vi "FPGA_DIOWriteOutputEnable.vi"(8 "error in (no error)":errorcluster, 10 "OutputEnable":u32, 11 "DIODeviceRef In":T1) -> (0 "error out":errorcluster, 3 "DIODeviceRef Out":T1)   [LabVIEW 2017]
uses:
  <vilib>/Rock Robotics/SystemInterfaces/DIO/FPGA_DIODevRef.ctl
  <vilib>/Rock Robotics/SystemInterfaces/System/FPGA_SystemFPGA Ref Global.vi
  <vilib>/Utility/error.llb/Error Cluster From Error Code.vi
  <vilib>/rvi/errors/niLvFpgaAdjustHostInterfaceError.vi
  <vilib>/rvi/interface/nirviReadWriteControl/nirviReadWriteControl.xnode
  <vilib>/Rock Robotics/SystemInterfaces/System/FPGA_SystemFRC FPGA Ref.ctl
  NiFpgaLv.dll
  <vilib>/rvi/interface/Simulation/niFpgaSimulationCallBeginRW.vi
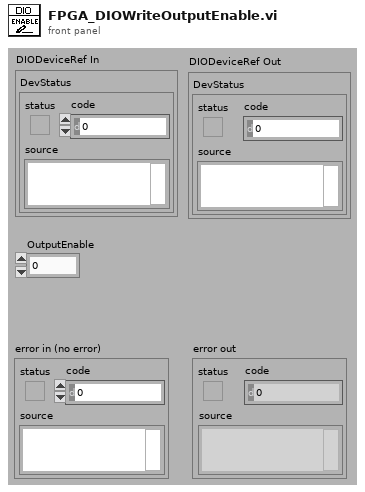
[diagram p1: front panel]
types:
  T1 = typedef "FPGA_DIODevRef.ctl" = cluster{"DevStatus":errorcluster}
  T2 = cluster{"Headers":fxp<+,10,10>, "SPIPort":fxp<+,5,5>, "Reserved":fxp<+,1,1>, "MXP":u16}
  T3 = typedef "FPGA_SystemFRC FPGA Ref.ctl" = refnum<k20>
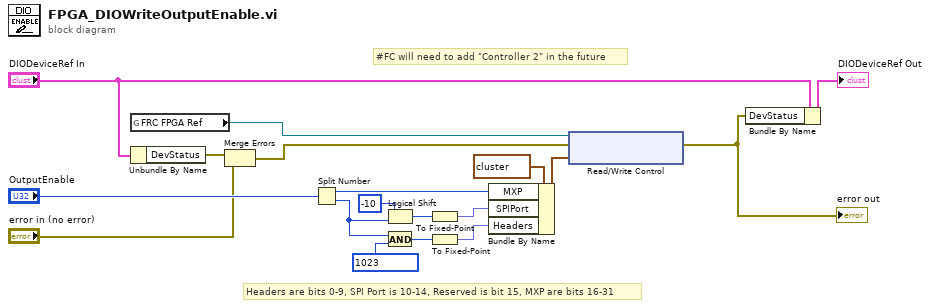
[diagram p0: block diagram]
diagram:
  # "Headers are bits 0-9, SPI Port is 10-14, Reserved is bit 15, MXP are bits 16-31"
  # "#FC will need to add \"Controller 2\" in the future"
  n1 = global read "FPGA_SystemFPGA Ref Global.vi" "FRC FPGA Ref"() -> (w16:T3)
  n2 = Unbundle By Name("DIODeviceRef In") -> ("DevStatus"=w15:errorcluster)
  n3 = Merge Errors(w15, "error in (no error)") -> (w14:errorcluster)
  n4 = Split Number(x="OutputEnable") -> (hi(x)=w11:u16, lo(x)=w9:u16)
  n5 = Logical Shift(y=i16 -10, x=w9) -> (x << y=w8:u16)
  n6 = And(x=w9, y=u16 1023) -> (x .and. y?=w6:u16)
  n7 = To Fixed-Point(number=w8) -> (fixed-point=w7:fxp<+,5,5>)  [unwired: 1 in]
  n8 = To Fixed-Point(number=w6) -> (fixed-point=w4:fxp<+,10,10>)  [unwired: 1 in]
  n9 = Bundle By Name(cluster=T2 {"Headers"=0.0, "SPIPort"=0.0, "Reserved"=0.0, "MXP"=0} ("DIO.OutputEnable"), "MXP"=w11, "SPIPort"=w7, "Headers"=w4) -> (w1:T2)
  n10 = xnode "Read/Write Control"("FPGA VI Reference In"=w16, "error in"=w14, "DIO.OutputEnable"=w1) -> ("error out"=w12:errorcluster)  [unwired: 1 out]
  "error out" <- w12
  n11 = Bundle By Name(cluster="DIODeviceRef In", "DevStatus"=w12) -> (→"DIODeviceRef Out":T1)
